vi "find empty cell (subvi).vi"(10 "Array":i32[][](array[ring]) items=["", "X", "0"]) -> (4 "Ничья":bool)   [LabVIEW 2017]
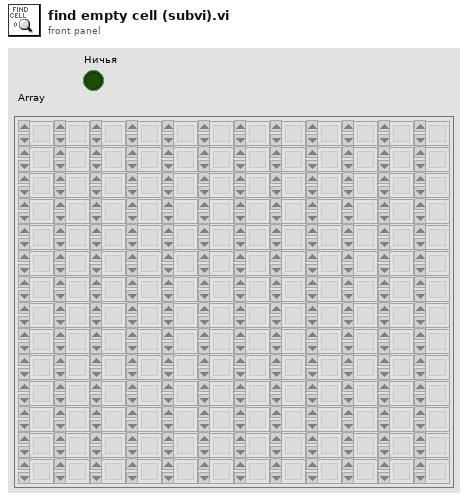
[diagram p1: front panel]
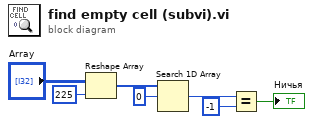
[diagram p0: block diagram]
diagram:
  n1 = Reshape Array("Array", 225 ("dimension size")) -> (w6:i32[])
  n2 = Search 1D Array(1D array=w6, element=0) -> (index of element=w4:i32)  [unwired: 1 in]
  n3 = Equal?(x=w4, y=-1) -> (x = y?=→"Ничья":bool)
